vi "laba6.vi"() -> ()   [LabVIEW 2021]
uses:
  <vilib>/Analysis/NI_AALPro.lvlib
panel:
  in  "Амплитуда":dbl(slide) scale=0.0..10.0
  out "ВЫХОД":i16[](graph)
  in  "max":dbl
  in  "min":dbl
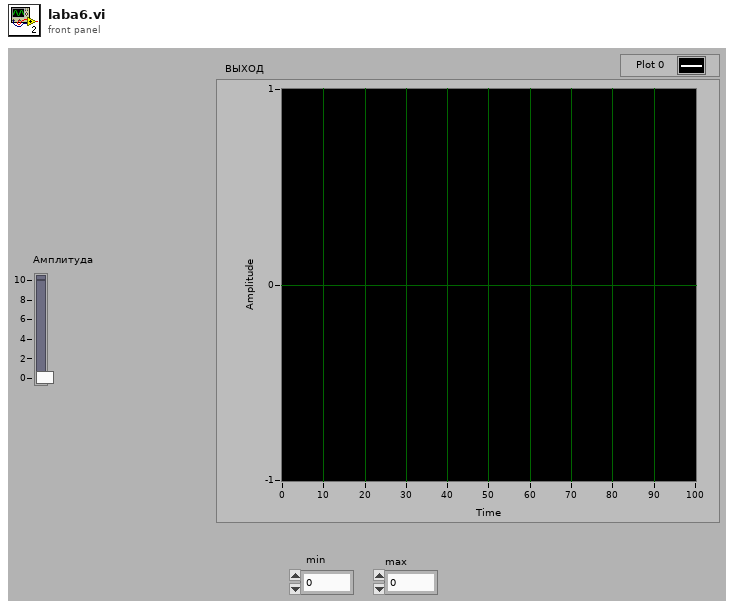
[diagram p1: front panel]
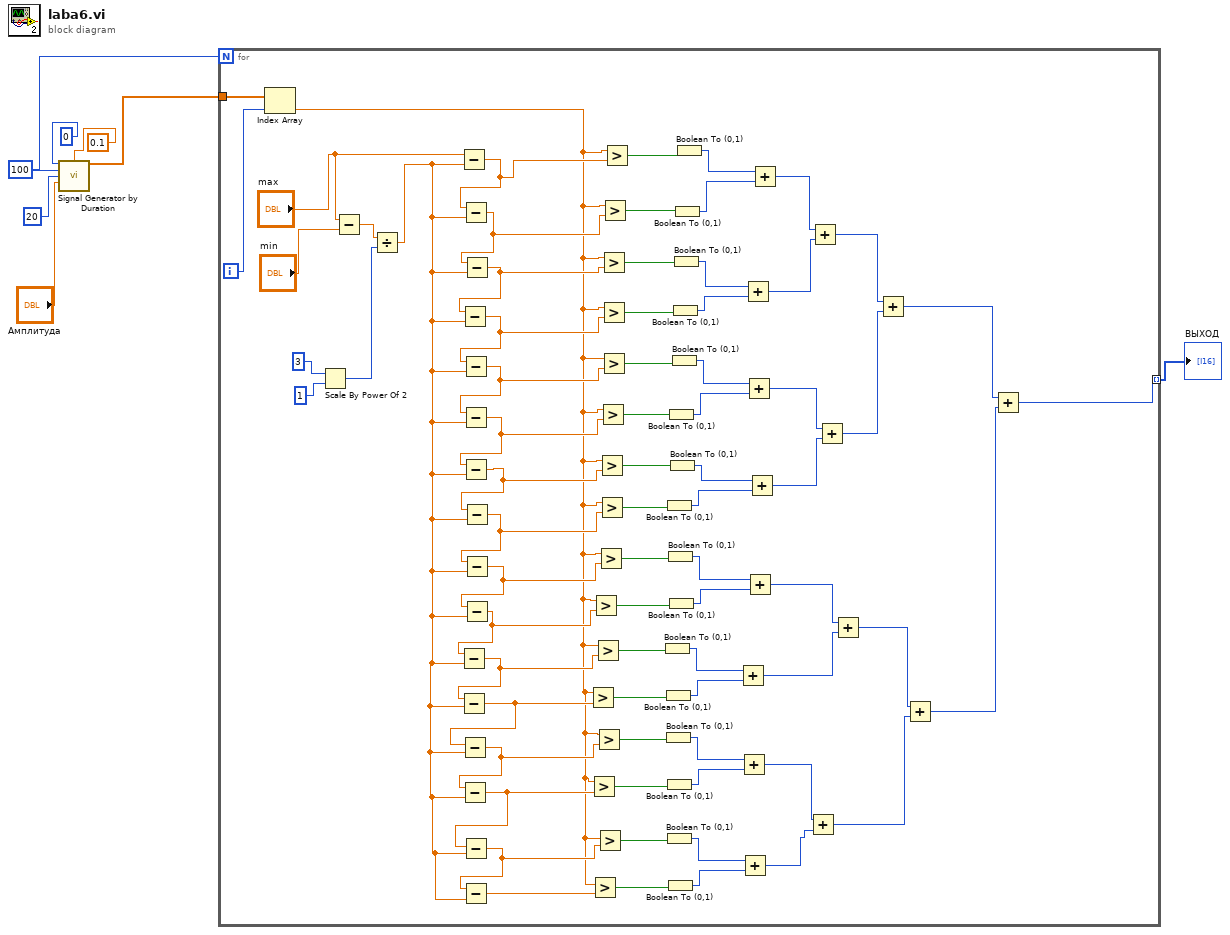
[diagram p0: block diagram]
diagram:
  w2 = 100
  n1 = call <vilib>:"Signal Generator by Duration.vi"("signal type"=0, "duration"=0.1, "# of samples"=w2, "frequency"=20, "amplitude"="Амплитуда") -> ("signal"=w3:dbl[])  [unwired: 2 in, 8 out]
  n2 = for {
    N: w2 -> [_]
    tunnel: [w30] -> w4 mode=indexing
    tunnel: w3 -> [w28]
    i -> [w29]
    n3 = Index Array(array=w28, index=w29) -> (element=w14:dbl)
    n4 = Scale By Power Of 2(n=3, x=1) -> (x*2^n=w76:i32)
    n5 = Subtract(x="max", y="min") -> (x-y=w74:dbl)
    n6 = Divide(x=w74, y=w76) -> (x/y=w8:dbl)
    n7 = Subtract(x="max", y=w8) -> (x-y=w78:dbl)
    n8 = Subtract(x=w78, y=w8) -> (x-y=w72:dbl)
    n9 = Subtract(x=w72, y=w8) -> (x-y=w71:dbl)
    n10 = Subtract(x=w71, y=w8) -> (x-y=w70:dbl)
    n11 = Subtract(x=w70, y=w8) -> (x-y=w69:dbl)
    n12 = Subtract(x=w69, y=w8) -> (x-y=w68:dbl)
    n13 = Subtract(x=w68, y=w8) -> (x-y=w67:dbl)
    n14 = Subtract(x=w67, y=w8) -> (x-y=w66:dbl)
    n15 = Subtract(x=w66, y=w8) -> (x-y=w44:dbl)
    n16 = Subtract(x=w44, y=w8) -> (x-y=w45:dbl)
    n17 = Subtract(x=w45, y=w8) -> (x-y=w46:dbl)
    n18 = Subtract(x=w46, y=w8) -> (x-y=w16:dbl)
    n19 = Subtract(x=w16, y=w8) -> (x-y=w25:dbl)
    n20 = Subtract(x=w25, y=w8) -> (x-y=w15:dbl)
    n21 = Subtract(x=w15, y=w8) -> (x-y=w19:dbl)
    n22 = Subtract(x=w19, y=w8) -> (x-y=w20:dbl)
    n23 = Greater?(x=w14, y=w16) -> (0:w47:bool)
    n24 = Greater?(x=w14, y=w15) -> (0:w26:bool)
    n25 = Greater?(x=w14, y=w20) -> (0:w21:bool)
    n26 = Greater?(x=w14, y=w45) -> (0:w49:bool)
    n27 = Greater?(x=w14, y=w46) -> (0:w48:bool)
    n28 = Greater?(x=w14, y=w25) -> (0:w27:bool)
    n29 = Greater?(x=w14, y=w19) -> (0:w22:bool)
    n30 = Greater?(x=w14, y=w44) -> (0:w58:bool)
    n31 = Greater?(x=w14, y=w67) -> (0:w60:bool)
    n32 = Greater?(x=w14, y=w66) -> (0:w59:bool)
    n33 = Greater?(x=w14, y=w68) -> (0:w61:bool)
    n34 = Greater?(x=w14, y=w71) -> (0:w64:bool)
    n35 = Greater?(x=w14, y=w70) -> (0:w63:bool)
    n36 = Greater?(x=w14, y=w69) -> (0:w62:bool)
    n37 = Greater?(x=w14, y=w72) -> (0:w65:bool)
    n38 = Greater?(x=w14, y=w78) -> (0:w77:bool)
    n39 = Boolean To (0,1)(Boolean=w48) -> (0, 1=w36:i16)
    n40 = Boolean To (0,1)(Boolean=w47) -> (0, 1=w35:i16)
    n41 = Boolean To (0,1)(Boolean=w27) -> (0, 1=w24:i16)
    n42 = Boolean To (0,1)(Boolean=w59) -> (0, 1=w50:i16)
    n43 = Boolean To (0,1)(Boolean=w26) -> (0, 1=w23:i16)
    n44 = Boolean To (0,1)(Boolean=w22) -> (0, 1=w18:i16)
    n45 = Boolean To (0,1)(Boolean=w58) -> (0, 1=w43:i16)
    n46 = Boolean To (0,1)(Boolean=w21) -> (0, 1=w17:i16)
    n47 = Boolean To (0,1)(Boolean=w61) -> (0, 1=w52:i16)
    n48 = Boolean To (0,1)(Boolean=w49) -> (0, 1=w42:i16)
    n49 = Boolean To (0,1)(Boolean=w60) -> (0, 1=w51:i16)
    n50 = Boolean To (0,1)(Boolean=w62) -> (0, 1=w53:i16)
    n51 = Boolean To (0,1)(Boolean=w63) -> (0, 1=w54:i16)
    n52 = Boolean To (0,1)(Boolean=w64) -> (0, 1=w55:i16)
    n53 = Boolean To (0,1)(Boolean=w65) -> (0, 1=w56:i16)
    n54 = Boolean To (0,1)(Boolean=w77) -> (0, 1=w57:i16)
    n55 = Add(x=w36, y=w35) -> (x+y=w34:i16)
    n56 = Add(x=w24, y=w23) -> (x+y=w13:i16)
    n57 = Add(x=w18, y=w17) -> (x+y=w12:i16)
    n58 = Add(x=w55, y=w54) -> (x+y=w40:i16)
    n59 = Add(x=w53, y=w52) -> (x+y=w39:i16)
    n60 = Add(x=w43, y=w42) -> (x+y=w37:i16)
    n61 = Add(x=w51, y=w50) -> (x+y=w38:i16)
    n62 = Add(x=w57, y=w56) -> (x+y=w41:i16)
    n63 = Add(x=w13, y=w12) -> (x+y=w11:i16)
    n64 = Add(x=w41, y=w40) -> (x+y=w33:i16)
    n65 = Add(x=w39, y=w38) -> (x+y=w32:i16)
    n66 = Add(x=w37, y=w34) -> (x+y=w10:i16)
    n67 = Add(x=w33, y=w32) -> (x+y=w31:i16)
    n68 = Add(x=w10, y=w11) -> (x+y=w9:i16)
    n69 = Add(x=w31, y=w9) -> (x+y=w30:i16)
  }
  "ВЫХОД" <- w4
